vi "IMAQ FPGA Camera Link Rising Edge Detect.vi"(10 "Input Valid":bool=TRUE, 11 "Input":bool) -> (3 "Rising Edge":bool)   [LabVIEW 2020]
doc: "This VI generates a single-cycle pulse each time there is a low-to-high transition on the input signal. This makes it easy to detect rising edges on signals."
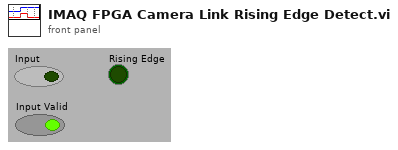
[diagram p1: front panel]
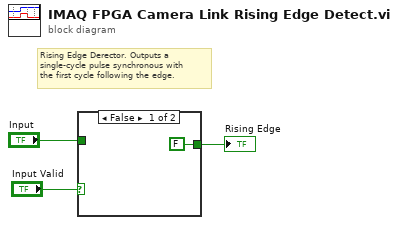
[diagram p0: block diagram]
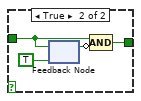
[diagram p2: hidden frame]
diagram:
  # "Rising Edge Derector. Outputs a\nsingle-cycle pulse synchronous with\nthe first cycle following the edge."
  n1 = case shown="False" "Input Valid" {
    tunnel: "Input" -> [_ w6]
    tunnel: [FALSE w5] -> w2
    frame False {
    }
    frame True {
      n2 = feedback #1(TRUE ("FV")) -> (w7:bool)
      n3 = feedback-in #1(w6) -> ()
      n4 = Compound Arithmetic op=AND(w6, invert w7) -> (w5:bool)
    }
  }
  "Rising Edge" <- w2
